vi "FB Core Mutate_1_1_2_0.vi"(8 "error in (no error)":errorcluster, 9 "Replies in":T1, 10 "Version":T3, 11 "Old State":T5) -> (0 "error out":errorcluster, 1 "Replies out":T1, 2 "Version Out":T3, 3 "New State":T5)   [LabVIEW 2020, in "FB Core.xnode"]
uses:
  <vilib>/functionblocks/FB Core/FB Core.xnode
  <vilib>/XNodeSupport/XNodeVariant.ctl
  <vilib>/XNodeSupport/XNodeVersion.ctl
  <vilib>/XNodeSupport/XNodeUShort.ctl
  <vilib>/XNodeSupport/XNodeStringArray.ctl
  <vilib>/XNodeSupport/XNodeString.ctl
  <vilib>/XNodeSupport/NI_XNodeSupport.lvlib
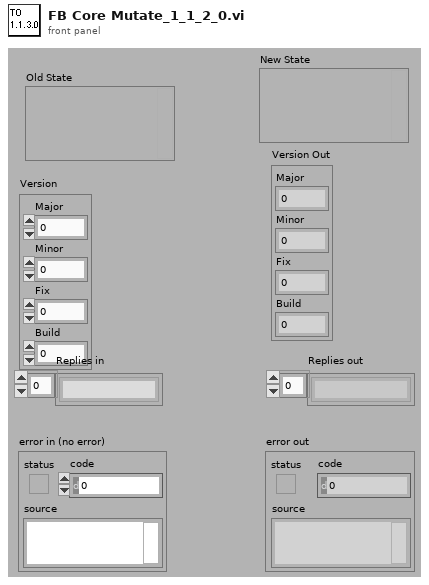
[diagram p1: front panel]
types:
  T1 = typedef "NI_XNodeSupport.lvlib/XNodeStringArray.ctl" = T2[]
  T2 = typedef "NI_XNodeSupport.lvlib/XNodeString.ctl" = string
  T3 = typedef "NI_XNodeSupport.lvlib/XNodeVersion.ctl" = cluster{"Major":T4, "Minor":T4, "Fix":T4, "Build":T4}
  T4 = typedef "NI_XNodeSupport.lvlib/XNodeUShort.ctl" = u16
  T5 = typedef "NI_XNodeSupport.lvlib/XNodeVariant.ctl" = variant
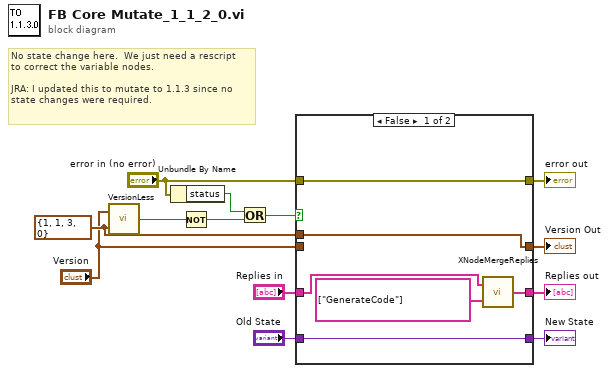
[diagram p0: block diagram]
diagram:
  w12 = T3 {"Major"=1, "Minor"=1, "Fix"=3, "Build"=0} ("y")
  # "No state change here.  We just need a rescript\nto correct the variable nodes.\n\nJRA: I updated this to mutate to 1.1.3 since no \nstate changes were required."
  n1 = call <vilib>:"VersionLess.vi"("y"=w12, "x"="Version") -> ("x < y?"=w13:bool)
  n2 = Unbundle By Name("error in (no error)") -> ("status"=w4:bool)
  n3 = Not(x=w13) -> (.not. x?=w3:bool)
  n4 = Or(x=w4, y=w3) -> (x .or. y?=w6:bool)
  n5 = case shown="False" w6 {
    tunnel: w12 -> [w19 _]
    tunnel: [w15 w23] -> w11
    tunnel: "Old State" -> [w15 w23]
    tunnel: [w19 w22] -> w9
    tunnel: "Version" -> [_ w22]
    tunnel: [w14 w21] -> w7
    tunnel: "error in (no error)" -> [w14 w21]
    tunnel: [w17 w20] -> w2
    tunnel: "Replies in" -> [w18 w20]
    frame False {
      n6 = call <vilib>:"XNodeMergeReplies.vi"("New Replies"=string[] ["GenerateCode"], "Old Replies"=w18) -> ("Merged Replies"=w17:string[])
    }
    frame True {
      # "Either there was an error in,\nor the version is not less than 1.0.0.6.\nPass input values out."
    }
  }
  "New State" <- w11
  "Version Out" <- w9
  "error out" <- w7
  "Replies out" <- w2
